vi "16 BIT MULTIRAM - 1 register.vi"(0 "Clock":bool, 1 "Hold":bool, 2 "Data In":bool[](array[boolean])=[FALSE, FALSE, FALSE, FALSE, FALSE, FALSE, FALSE, FALSE, FALSE, FALSE, FALSE, FALSE, FALSE, FALSE, FALSE, FALSE], 3 "Address of this register":bool[](array[boolean])=[FALSE, FALSE, FALSE, FALSE, FALSE, FALSE, FALSE, FALSE, FALSE, FALSE, FALSE, FALSE, FALSE, FALSE, FALSE, FALSE], 4 "Destination Address In":bool[](array[boolean])=[FALSE, FALSE, FALSE, FALSE, FALSE, FALSE, FALSE, FALSE, FALSE, FALSE, FALSE, FALSE, FALSE, FALSE, FALSE, FALSE], 5 "Address'":bool[][](array[boolean])) -> (6 "z":bool[](array[boolean]), 7 "Destination Address Out":bool[](array[boolean]), 8 "Operational?":bool)   [LabVIEW 2012]
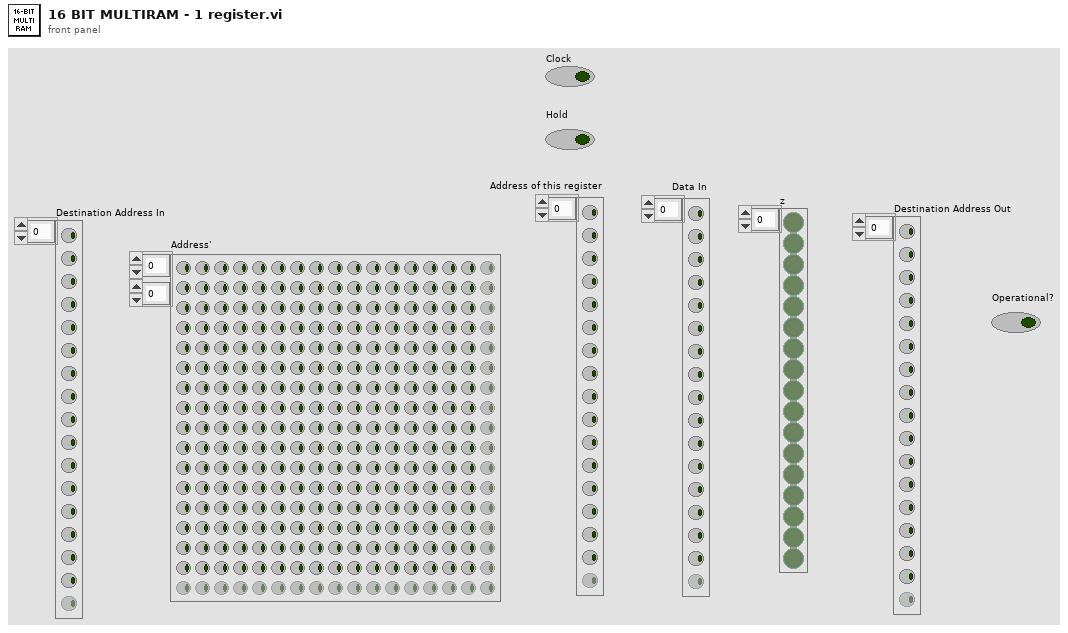
[diagram p1: front panel]
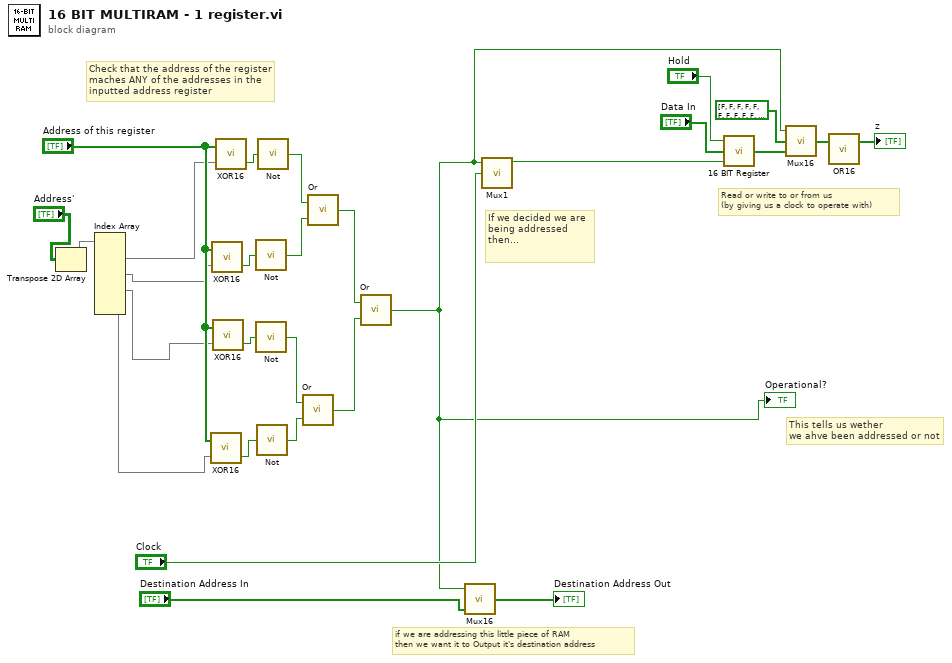
[diagram p0: block diagram]
diagram:
  # "This tells us wether\nwe ahve been addressed or not"
  # "Read or write to or from us\n(by giving us a clock to operate with)"
  # "If we decided we are being addressed then..."
  # "Check that the address of the register\nmaches ANY of the addresses in the\ninputted address register"
  # "if we are addressing this little piece of RAM\nthen we want it to Output it's destination address"
  n1 = Transpose 2D Array(2D array="Address'") -> (transposed array=w16:bool[][])
  n2 = Index Array(array=w16) -> (element #1=w14:bool[], element #2=w5:bool[], element #3=w4:bool[], element #4=w3:bool[])  [unwired: 8 in]
  n3 = call "XOR16.vi"("B"=w3, "A"="Address of this register") -> ("compound"=w11:bool)  [unwired: 1 out]
  n4 = call "XOR16.vi"("B"=w5, "A"="Address of this register") -> ("compound"=w10:bool)  [unwired: 1 out]
  n5 = call "XOR16.vi"("B"=w4, "A"="Address of this register") -> ("compound"=w12:bool)  [unwired: 1 out]
  n6 = call "XOR16.vi"("B"=w14, "A"="Address of this register") -> ("compound"=w13:bool)  [unwired: 1 out]
  n7 = call "Not.vi"("In"=w10) -> ("Out"=w8:bool)
  n8 = call "Not.vi"("In"=w12) -> ("Out"=w7:bool)
  n9 = call "Not.vi"("In"=w11) -> ("Out"=w6:bool)
  n10 = call "Not.vi"("In"=w13) -> ("Out"=w9:bool)
  n11 = call "Or.vi"("b"=w6, "a"=w7) -> ("x"=w20:bool)
  n12 = call "Or.vi"("b"=w8, "a"=w9) -> ("x"=w19:bool)
  n13 = call "Or.vi"("b"=w20, "a"=w19) -> ("x"=w1:bool)
  "Operational?" <- w1
  n14 = call "Mux16.vi"("B"="Destination Address In", "s0"=w1) -> ("z"=→"Destination Address Out":bool[])  [unwired: 1 in]
  n15 = call "Mux1.vi"("A"="Clock", "s0"=w1) -> ("z"=w22:bool)  [unwired: 1 in]
  n16 = call "16 BIT Register.vi"("Clock"=w22, "Data In"="Data In", "Hold"="Hold") -> ("Data Out"=w26:bool[])
  n17 = call "Mux16.vi"("B"=w26, "A"=bool[] [FALSE, FALSE, FALSE, FALSE, FALSE, FALSE, FALSE, FALSE, FALSE, FALSE, FALSE, FALSE, FALSE, FALSE, FALSE, FALSE] ("B"), "s0"=w1) -> ("z"=w24:bool[])
  n18 = call "OR16.vi"("A"=w24) -> ("z"=→"z":bool[])  [unwired: 1 in, 1 out]
